vi "Search and Replace String, Substring Part 2.vi"() -> ()   [LabVIEW 2020]
panel:
  out "Search and Replace String":string
  out "replaced substring":string
  out "result string":string
  in  "string":string
  in  "substring (\"\")":string
  # "Part 2"
  # "Search and Replace String \n                  &\n             Substring"
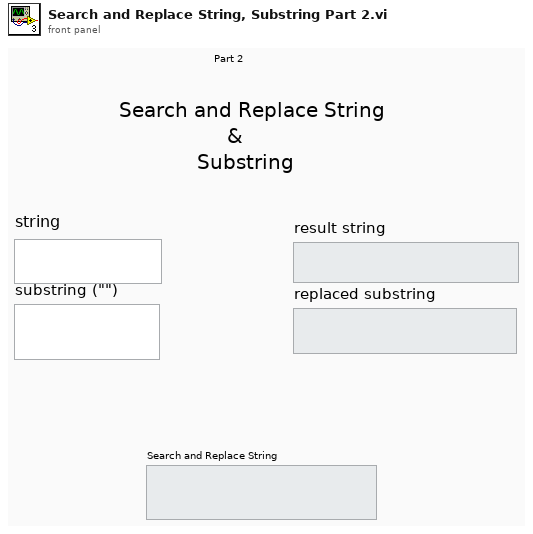
[diagram p1: front panel]
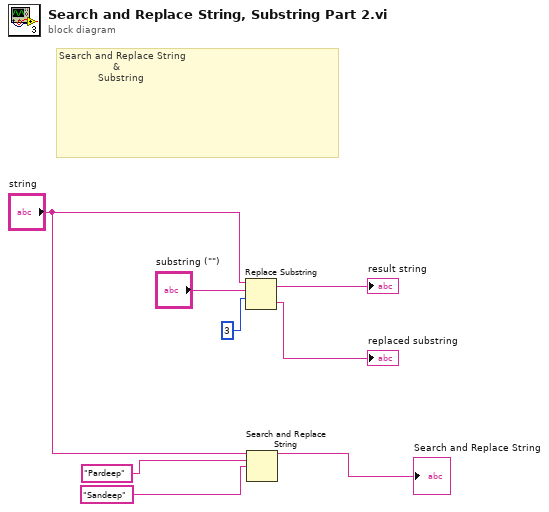
[diagram p0: block diagram]
diagram:
  # "Search and Replace String \n                  &\n             Substring"
  n1 = Replace Substring(3:3 ("offset (0)"), 4:"substring (\"\")", 5:"string") -> (0:→"replaced substring":string, 1:→"result string":string)  [unwired: 1 in]
  n2 = Search and Replace String(input string="string", search string="Pardeep", replace string="Sandeep" ("replace string (\"\")")) -> (result string=→"Search and Replace String":string)  [unwired: 5 in, 3 out]
